vi "SNR.vi"(10 "Array":cdb[](array[numeric]), 11 "OFDM":cdb[](array[numeric])) -> (2 "Numeric":dbl)   [LabVIEW 2018]
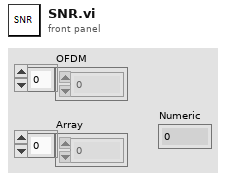
[diagram p1: front panel]
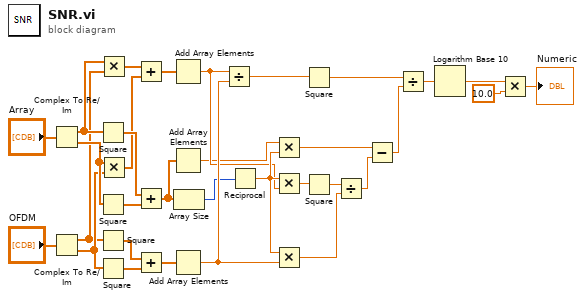
[diagram p0: block diagram]
diagram:
  n1 = Complex To Re/Im(x + iy="Array") -> (x=w11:dbl[], y=w12:dbl[])
  n2 = Complex To Re/Im(x + iy="OFDM") -> (x=w4:dbl[], y=w5:dbl[])
  n3 = Square(x=w11) -> (x^2=w9:dbl[])
  n4 = Square(x=w12) -> (x^2=w10:dbl[])
  n5 = Square(x=w4) -> (x^2=w6:dbl[])
  n6 = Square(x=w5) -> (x^2=w7:dbl[])
  n7 = Multiply(x=w11, y=w4) -> (x*y=w1:dbl[])
  n8 = Multiply(x=w12, y=w5) -> (x*y=w2:dbl[])
  n9 = Add(x=w1, y=w2) -> (x+y=w3:dbl[])
  n10 = Add(x=w9, y=w10) -> (x+y=w13:dbl[])
  n11 = Add(x=w6, y=w7) -> (x+y=w8:dbl[])
  n12 = Add Array Elements(numeric array=w3) -> (sum=w17:dbl)
  n13 = Add Array Elements(numeric array=w13) -> (sum=w16:dbl)
  n14 = Add Array Elements(numeric array=w8) -> (sum=w21:dbl)
  n15 = Array Size(array=w13) -> (size(s)=w14:i32)
  n16 = Divide(x=w17, y=w21) -> (x/y=w15:dbl)
  n17 = Reciprocal(x=w14) -> (1/x=w20:dbl)
  n18 = Multiply(x=w16, y=w20) -> (x*y=w23:dbl)
  n19 = Multiply(x=w20, y=w17) -> (x*y=w18:dbl)
  n20 = Multiply(x=w20, y=w21) -> (x*y=w22:dbl)
  n21 = Square(x=w15) -> (x^2=w26:dbl)
  n22 = Square(x=w18) -> (x^2=w19:dbl)
  n23 = Divide(x=w19, y=w22) -> (x/y=w24:dbl)
  n24 = Subtract(x=w23, y=w24) -> (x-y=w25:dbl)
  n25 = Divide(x=w26, y=w25) -> (x/y=w27:dbl)
  n26 = Logarithm Base 10(1:w27) -> (0:w28:dbl)
  n27 = Multiply(x=w28, y=10.0) -> (x*y=→"Numeric":dbl)
